vi "Tag Names.vi"(11 "Process Name":string) -> (2 "Flow Tags":T1, 4 "All Boolean Tags":string[](array[string]), 5 "All  Numeric Tags":string[](array[string]))   [LabVIEW 2018, in "Flow Module.lvlib" / "Flow Module Engine.lvlib"]
uses:
  Flow Module Engine.lvlib
  Bronkhorst M14 Flow Meter/Tag Cluster.ctl
  Flow Module.lvlib
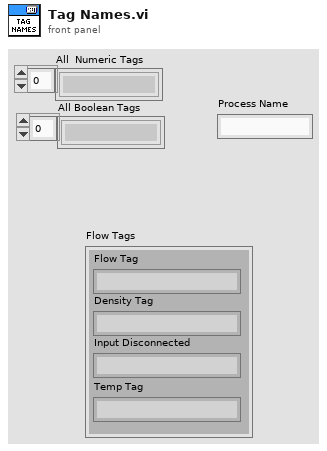
[diagram p1: front panel]
types:
  T1 = typedef "Flow Module.lvlib/Tag Cluster.ctl" = cluster{"Flow Tag":string, "Input Disconnected":string, "Density Tag":string, "Temp Tag":string}
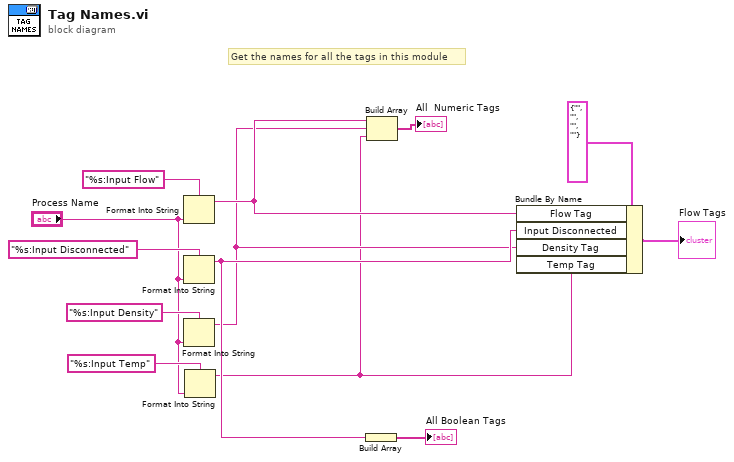
[diagram p0: block diagram]
diagram:
  # "Get the names for all the tags in this module"
  n1 = Format Into String(format string="%s:Input Flow", "Process Name") -> (resulting string=w9:string)  [unwired: 2 in, 1 out]
  n2 = Format Into String(format string="%s:Input Disconnected", "Process Name") -> (resulting string=w8:string)  [unwired: 2 in, 1 out]
  n3 = Format Into String(format string="%s:Input Density", "Process Name") -> (resulting string=w5:string)  [unwired: 2 in, 1 out]
  n4 = Format Into String(format string="%s:Input Temp", "Process Name") -> (resulting string=w1:string)  [unwired: 2 in, 1 out]
  n5 = Build Array(w8) -> (→"All Boolean Tags":string[])
  n6 = Build Array(w9, w5, w1) -> (→"All  Numeric Tags":string[])
  n7 = Bundle By Name(cluster=T1 {"Flow Tag"="", "Input Disconnected"="", "Density Tag"="", "Temp Tag"=""} ("Flow Tags 2"), "Flow Tag"=w9, "Input Disconnected"=w8, "Density Tag"=w5, "Temp Tag"=w1) -> (→"Flow Tags":T1)
